vi "TL2100LAB06.vi"() -> ()   [LabVIEW 2020]
panel:
  out "Vin":dbl(slide) scale=-1.2..1.8 scale format="%.1g"
  out "AtoD":i16 format="%04x"
  out "Thermometer":dbl(slide) scale=10.0..40.0 scale format="%.1g"
  out "Temperature Chart":dbl(graph)
  in  "?":bool
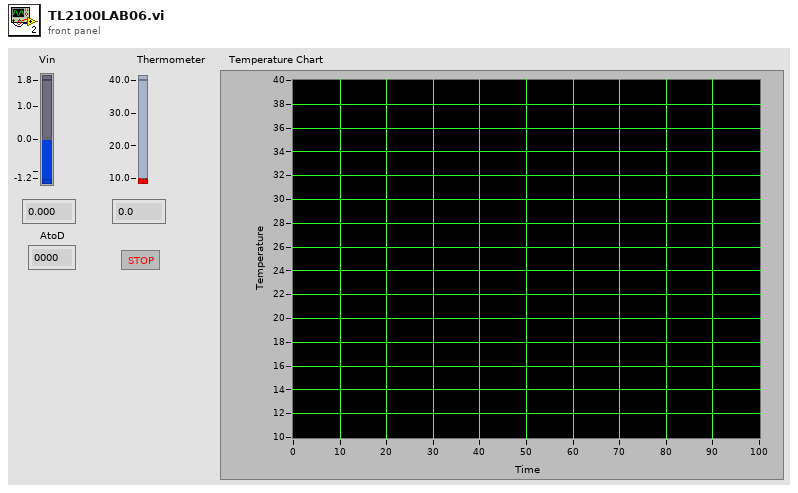
[diagram p1: front panel]
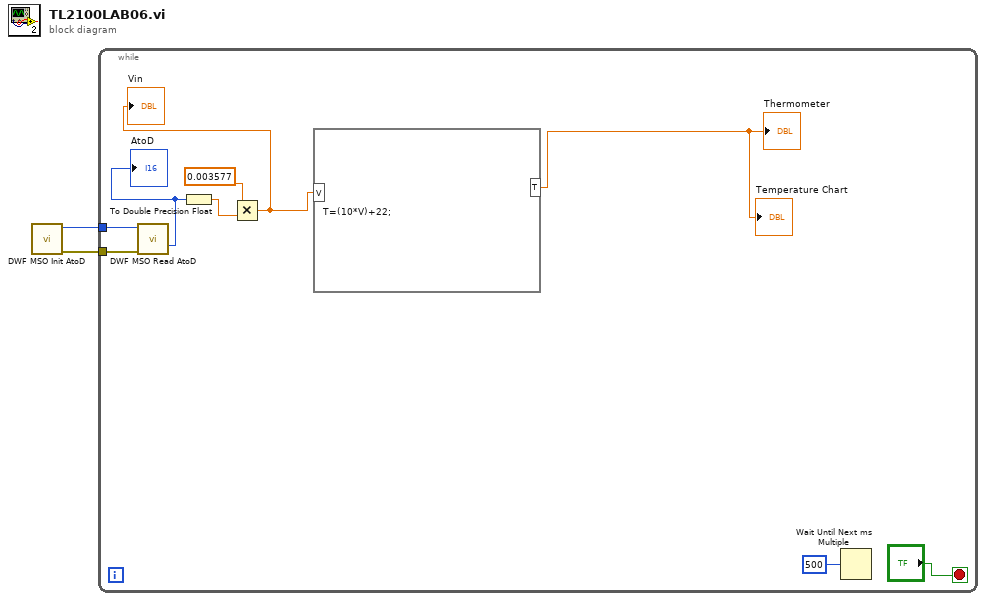
[diagram p0: block diagram]
diagram:
  n1 = call "DWF MSO Init AtoD.vi"() -> ("Error Out"=w1:errorcluster, "Instrument Handle Out"=w2:u32)  [unwired: 10 in]
  n2 = while {
    tunnel: w2 -> [w9]
    tunnel: w1 -> [w8]
    stop <- "?" stop-if-true
    n3 = call "DWF MSO Read AtoD.vi"("Instrument Handle In AtoD"=w9, "Error In"=w8) -> ("AtoD"=w5:i16)  [unwired: 12 in, 1 out]
    "AtoD" <- w5
    n4 = To Double Precision Float(number=w5) -> (double precision float=w6:dbl)
    n5 = Multiply(x=0.003577, y=w6) -> (x*y=w3:dbl)
    "Vin" <- w3
    n6 = formula code="T=(10*V)+22;"("V"=w3) -> ("T"=→"Temperature Chart" →"Thermometer":dbl)
    n7 = Wait Until Next ms Multiple(millisecond multiple=500) -> ()  [unwired: 1 out]
  }
